vi "Init.vi"(11 "error in (no error)":errorcluster) -> (4 "FPGA API out":refnum<class "FPGA API Concrete.lvclass">, 15 "error out":errorcluster)   [LabVIEW 2019, in "FPGA API Concrete.lvclass"]
uses:
  FPGA API Concrete.lvclass
  FPGA/TypeDef/DO index.ctl
  FPGA API Concrete.lvclass/FPGA API Concrete.ctl
  <vilib>/FPGAPlugInAG/cRIO-9035/niLvFpga_Open_cRIO-9035.vi
  <vilib>/rvi/interface/common/dynamic/niFpgaDynamicAddResources.vi
  <vilib>/rvi/interface/common/niFpgaWaitOnOcc.vi
  <vilib>/Utility/error.llb/Error Cluster From Error Code.vi
  <vilib>/rvi/interface/nirviOpenFPGA/nirviOpenFPGA.xnode
  FPGA Bitfiles/MAIN_FPGA.lvbitx
  <vilib>/rvi/interface/nirviMethod/nirviMethod.xnode
  <vilib>/rvi/errors/niLvFpgaMergeErrorWithErrorCode.vi
  <vilib>/FPGAPlugInAG/Dynamic/niLvFpga_ConfigureFifo_Dynamic.vi
  <vilib>/FPGAPlugInAG/Dynamic/niLvFpga_StartFifo_Dynamic.vi
  FPGA Ref.ctl
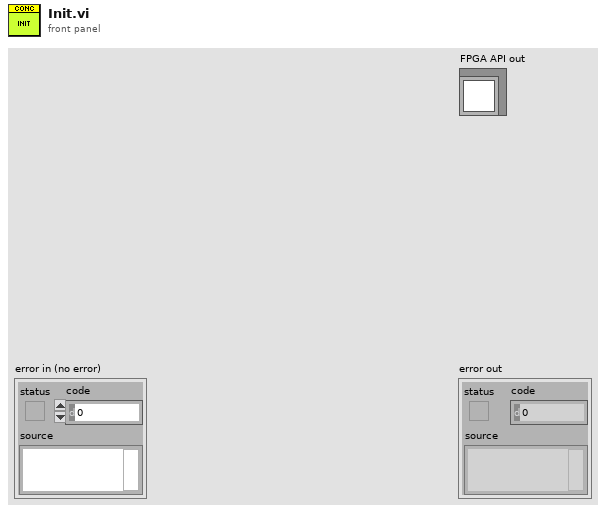
[diagram p1: front panel]
types:
  T1 = typedef "DO index.ctl" = u8
  T2 = typedef "FPGA API Concrete.lvclass/FPGA Ref.ctl" = refnum<k20>
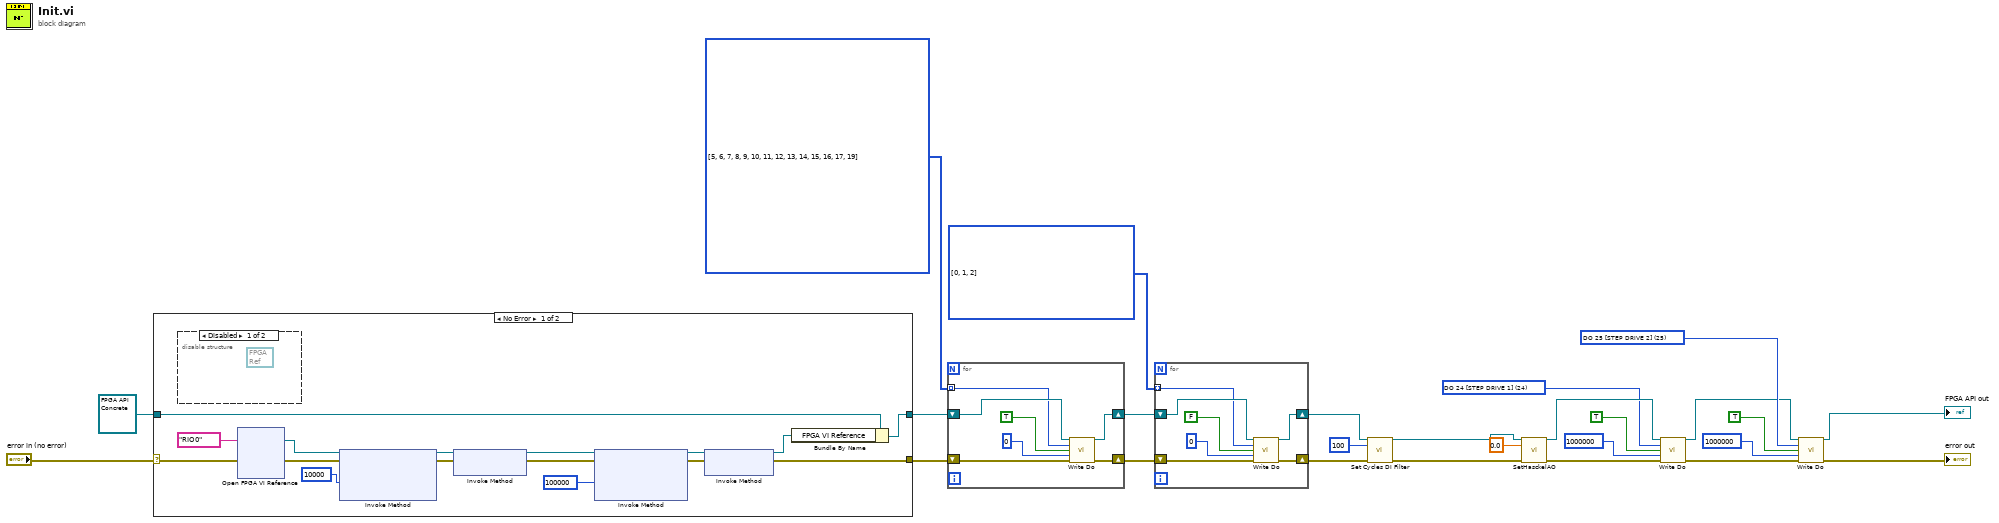
[diagram p0: block diagram]
diagram:
  w9 = T1[] [0, 1, 2] items=["DO 0 [KP1] [M12]", "DO 1 [ON KP2] [M21]", "DO 2 [ON KP3] [M24]", "DO 3 [WATER Y18.1 [DO3]]", "DO 4 [WATER Y18.2 [DO4]]", "DO 5 [KP6 Y29.1 33.7]", "DO 6 [KP7 Y29.2 33.8]", "DO 7 [KP8 Y29.3 33.9]", "DO 8 [KP9 Y29.4  33.12]", "DO 9 [KP10 Y29.5 33.1]", "DO 10 [KP11 Y29.6 33.2]", "DO 11 [KP12 Y29.7  33.13]", "DO 12 [KP13 Y29.8  33.11]", "DO 13 [KP14 Y29.9 33.10]", "DO 14 [KP15 Y29.10  33.6]", "DO 15 [KP16 Y29.11  33.5]", "DO 16 [KP17 Y29.12  33.4]", "DO 17 [KP18 Y29.13 33.3]", "DO 18 [AIR KP19]", "DO 19 [STEP DRIVE EN KP20]", "DO 20 [KP21 Y44.1 OPEN]", "DO 21 [ KP22 Y44.1 CLOSE]", "DO 22 [ KP23 Y44.2 OPEN]", "DO 23", "DO 24 [STEP DRIVE 1]", "DO 25 [STEP DRIVE 2]"] ("#DO")
  w15 = T1 25 items=["DO 0 [KP1 [DO 0]]", "DO 1 [ON KP2 [DO 1]]", "DO 2 [ON KP3 [DO 2]]", "DO 3 [WATER Y18.1 [DO3]]", "DO 4 [WATER Y18.2 [DO4]]", "DO 5 [KP6 Y29.1 33.7]", "DO 6 [KP7 Y29.2 33.8]", "DO 7 [KP8 Y29.3 33.9]", "DO 8 [KP9 Y29.4  33.12]", "DO 9 [KP10 Y29.5 33.1]", "DO 10 [KP11 Y29.6 33.2]", "DO 11 [KP12 Y29.7  33.13]", "DO 12 [KP13 Y29.8  33.11]", "DO 13 [KP14 Y29.9 33.10]", "DO 14 [KP15 Y29.10  33.6]", "DO 15 [KP16 Y29.11  33.5]", "DO 16 [KP17 Y29.12  33.4]", "DO 17 [KP18 Y29.13 33.3]", "DO 18 [AIR KP19]", "DO 19 [STEP DRIVE EN KP20]", "DO 20 [KP21 Y44.1 OPEN]", "DO 21 [ KP22 Y44.1 CLOSE]", "DO 22 [ KP23 Y44.2 OPEN]", "DO 23", "DO 24 [STEP DRIVE 1]", "DO 25 [STEP DRIVE 2]"] ("#DO")
  w18 = T1 24 items=["DO 0 [KP1 [DO 0]]", "DO 1 [ON KP2 [DO 1]]", "DO 2 [ON KP3 [DO 2]]", "DO 3 [WATER Y18.1 [DO3]]", "DO 4 [WATER Y18.2 [DO4]]", "DO 5 [KP6 Y29.1 33.7]", "DO 6 [KP7 Y29.2 33.8]", "DO 7 [KP8 Y29.3 33.9]", "DO 8 [KP9 Y29.4  33.12]", "DO 9 [KP10 Y29.5 33.1]", "DO 10 [KP11 Y29.6 33.2]", "DO 11 [KP12 Y29.7  33.13]", "DO 12 [KP13 Y29.8  33.11]", "DO 13 [KP14 Y29.9 33.10]", "DO 14 [KP15 Y29.10  33.6]", "DO 15 [KP16 Y29.11  33.5]", "DO 16 [KP17 Y29.12  33.4]", "DO 17 [KP18 Y29.13 33.3]", "DO 18 [AIR KP19]", "DO 19 [STEP DRIVE EN KP20]", "DO 20 [KP21 Y44.1 OPEN]", "DO 21 [ KP22 Y44.1 CLOSE]", "DO 22 [ KP23 Y44.2 OPEN]", "DO 23", "DO 24 [STEP DRIVE 1]", "DO 25 [STEP DRIVE 2]"] ("#DO")
  w21 = T1[] [5, 6, 7, 8, 9, 10, 11, 12, 13, 14, 15, 16, 17, 19] items=["DO 0 [KP1 [DO 0]]", "DO 1 [ON KP2 [DO 1]]", "DO 2 [ON KP3 [DO 2]]", "DO 3 [WATER Y18.1 [DO3]]", "DO 4 [WATER Y18.2 [DO4]]", "DO 5 [KP6 Y29.1 33.7]", "DO 6 [KP7 Y29.2 33.8]", "DO 7 [KP8 Y29.3 33.9]", "DO 8 [KP9 Y29.4  33.12]", "DO 9 [KP10 Y29.5 33.1]", "DO 10 [KP11 Y29.6 33.2]", "DO 11 [KP12 Y29.7  33.13]", "DO 12 [KP13 Y29.8  33.11]", "DO 13 [KP14 Y29.9 33.10]", "DO 14 [KP15 Y29.10  33.6]", "DO 15 [KP16 Y29.11  33.5]", "DO 16 [KP17 Y29.12  33.4]", "DO 17 [KP18 Y29.13 33.3]", "DO 18 [AIR KP19]", "DO 19 [STEP DRIVE EN KP20]", "DO 20 [KP21 Y44.1 OPEN]", "DO 21 [ KP22 Y44.1 CLOSE]", "DO 22 [ KP23 Y44.2 OPEN]", "DO 23", "DO 24 [STEP DRIVE 1]", "DO 25 [STEP DRIVE 2]"] ("#DO")
  n1 = case shown="No Error" "error in (no error)" {
    selector: "error in (no error)" -> [w36 w44]
    tunnel: [w27 w44] -> w22
    tunnel: [w34 w43] -> w23
    tunnel: refnum<class "FPGA API Concrete.lvclass"> refnum ("FPGA API in") -> [w42 w43]
    frame No Error {
      n2 = disable-structure shown="Disabled" {
        frame Disabled {
          (unwired) T2 refnum ("FPGA VI Reference")
        }
        frame Enabled {
        }
      }
      n3 = xnode "Open FPGA VI Reference"("error in"=w36, "resource name"=tag "RIO0") -> ("FPGA VI Reference Out"=w41:refnum<k20>, "error out"=w37:errorcluster)
      n4 = xnode "Invoke Method"("FPGA VI Reference In"=w41, "error in"=w37, "Requested Depth"=u32 10000) -> ("FPGA VI Reference Out"=w39:refnum<k20>, "error out"=w38:errorcluster)  [unwired: 1 out]
      n5 = xnode "Invoke Method"("FPGA VI Reference In"=w39, "error in"=w38) -> ("FPGA VI Reference Out"=w30:refnum<k20>, "error out"=w29:errorcluster)
      n6 = xnode "Invoke Method"("FPGA VI Reference In"=w30, "error in"=w29, "Requested Depth"=u32 100000) -> ("FPGA VI Reference Out"=w33:refnum<k20>, "error out"=w32:errorcluster)  [unwired: 1 out]
      n7 = xnode "Invoke Method"("FPGA VI Reference In"=w33, "error in"=w32) -> ("FPGA VI Reference Out"=w28:refnum<k20>, "error out"=w27:errorcluster)
      n8 = Bundle By Name(cluster=w42, "FPGA VI Reference"=w28) -> (w34:refnum<class "FPGA API Concrete.lvclass">)
    }
    frame Error {
    }
  }
  n9 = for {
    tunnel: w21 -> [w47] mode=indexing
    shift-right: [w50] -> w8
    shift-left: w23 -> [w51]
    shift-right: [w49] -> w6
    shift-left: w22 -> [w48]
    n10 = call-dynamic "Write Do.vi"("FPGA API in"=w51, "#DO"=w47, "value"=TRUE, "Time uSec"=u32 0, "error in (no error)"=w48) -> ("FPGA API out"=w50:refnum<class "FPGA API Concrete.lvclass">, "error out"=w49:errorcluster)  [unwired: 9 in]
  }
  n11 = for {
    tunnel: w9 -> [w54] mode=indexing
    shift-right: [w57] -> w7
    shift-left: w8 -> [w58]
    shift-right: [w56] -> w5
    shift-left: w6 -> [w55]
    n12 = call-dynamic "Write Do.vi"("FPGA API in"=w58, "#DO"=w54, "value"=FALSE, "Time uSec"=u32 0, "error in (no error)"=w55) -> ("FPGA API out"=w57:refnum<class "FPGA API Concrete.lvclass">, "error out"=w56:errorcluster)  [unwired: 9 in]
  }
  n13 = call "Set Cycles DI Filter.vi"("FPGA API in"=w7, "Cycles to Filter"=u16 100, "error in (no error)"=w5) -> ("FPGA API out"=w2:refnum<class "FPGA API Concrete.lvclass">, "error out"=w1:errorcluster)  [unwired: 11 in]
  n14 = call-dynamic "SetHasckelAO.vi"("FPGA API in"=w2, "Haskel in"=0.0, "error in (no error)"=w1) -> ("FPGA API out"=w19:refnum<class "FPGA API Concrete.lvclass">, "error out"=w11:errorcluster)  [unwired: 11 in]
  n15 = call-dynamic "Write Do.vi"("FPGA API in"=w19, "#DO"=w18, "value"=TRUE, "Time uSec"=u32 1000000, "error in (no error)"=w11) -> ("FPGA API out"=w14:refnum<class "FPGA API Concrete.lvclass">, "error out"=w10:errorcluster)  [unwired: 9 in]
  n16 = call-dynamic "Write Do.vi"("FPGA API in"=w14, "#DO"=w15, "value"=TRUE, "Time uSec"=u32 1000000, "error in (no error)"=w10) -> ("FPGA API out"=→"FPGA API out":refnum<class "FPGA API Concrete.lvclass">, "error out"=→"error out":errorcluster)  [unwired: 9 in]
